vi "ReadArrayDouble(DBL).vi"(8 "error in (no error)":errorcluster, 9 "Elements (-1 = auto)":i32, 10 "variableName":string, 11 "TCatAdsNet in":refnum<class "AdsNET.lvclass">) -> (0 "error out":errorcluster, 2 "Values (DBL)":dbl[](array[numeric]), 3 "TCatAdsNet out":refnum<class "AdsNET.lvclass">)   [LabVIEW 2016, in "TCatAdsNet.lvlib" / "AdsNET.lvclass"]
uses:
  AdsNET.lvclass
  AdsNET.lvclass/AdsNET.ctl
  C:/Users/Maurizio/Projects/twincat-lv-ads-library/TCatAdsNet Library/TwinCAT.Ads.dll
  TwinCAT.Ads.dll
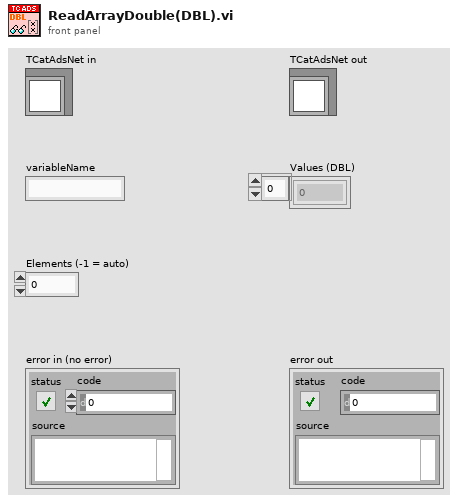
[diagram p1: front panel]
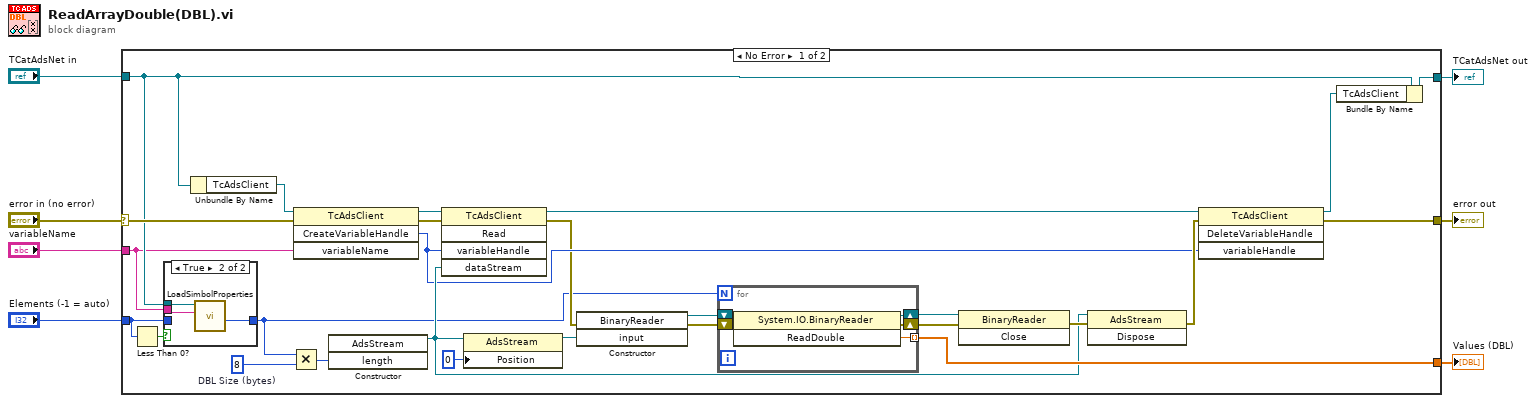
[diagram p0: block diagram]
diagram:
  n1 = case shown="No Error" "error in (no error)" {
    selector: "error in (no error)" -> [w13 w43]
    tunnel: [w27 _] -> w7
    tunnel: "variableName" -> [w10 _]
    tunnel: "Elements (-1 = auto)" -> [w9 _]
    tunnel: [w16 w44] -> w4
    tunnel: [w14 w43] -> w3
    tunnel: "TCatAdsNet in" -> [w11 w44]
    frame No Error {
      w32 = 8  # DBL Size (bytes)
      n2 = Less Than 0?(x=w9) -> (x < 0?=w8:bool)
      n3 = case shown="True" w8 {
        tunnel: w9 -> [w35 _]
        tunnel: [w35 w38] -> w12
        tunnel: w11 -> [_ w37]
        tunnel: w10 -> [_ w36]
        frame False {
        }
        frame True {
          n4 = call "LoadSimbolProperties.vi"("name"=w36, "TCatAdsNet in"=w37) -> ("Elements"=w38:i32)  [unwired: 6 in, 3 out]
        }
      }
      n5 = Unbundle By Name(w11) -> ("TcAdsClient"=w17:refnum<k24>)
      n6 = Multiply ("Multiplizieren")(x=w12, y=w32) -> (x*y=w31:i32)
      n7 = invoke class="TcAdsClient" method="CreateVariableHandle"(reference=w17, error in=w13, "variableName"=w10) -> (reference out=w34:refnum<k24>, error out=w33:errorcluster, "CreateVariableHandle"=w19:i32)  [unwired: 1 in, 1 out]
      n8 = constructor class="AdsStream" ("Konstruktorknoten")("length"=w31) -> (reference out=w21:refnum<k24>)  [unwired: 3 in, 3 out]
      n9 = invoke class="TcAdsClient" method="Read"(reference=w34, error in=w33, "variableHandle"=w19, "dataStream"=w21) -> (reference out=w22:refnum<k24>, error out=w18:errorcluster)  [unwired: 1 in, 3 out]
      n10 = property class="AdsStream"(reference=w21, "Position"=i64 0) -> (reference out=w29:refnum<k24>)  [unwired: 1 in, 1 out]
      n11 = constructor class="BinaryReader"(error in=w18, "input"=w29) -> (reference out=w28:refnum<k24>, error out=w25:errorcluster)  [unwired: 2 in, 2 out]
      n12 = for {
        N: w12 -> [_]
        tunnel: [w41] -> w27 mode=indexing
        shift-right: [w40] -> w26
        shift-left: w28 -> [w42]
        shift-right: [w39] -> w24
        shift-left: w25 -> [_]
        n13 = invoke class="System.IO.BinaryReader" method="ReadDouble"(reference=w42) -> (reference out=w40:refnum<k24>, error out=w39:errorcluster, "ReadDouble"=w41:dbl)  [unwired: 2 in]
      }
      n14 = invoke class="BinaryReader" method="Close"(reference=w26, error in=w24) -> (error out=w23:errorcluster)  [unwired: 1 in, 2 out]
      n15 = invoke class="AdsStream" method="Dispose"(reference=w21, error in=w23) -> (error out=w20:errorcluster)  [unwired: 1 in, 2 out]
      n16 = invoke class="TcAdsClient" method="DeleteVariableHandle"(reference=w22, error in=w20, "variableHandle"=w19) -> (reference out=w15:refnum<k24>, error out=w14:errorcluster)  [unwired: 1 in, 2 out]
      n17 = Bundle By Name(cluster=w11, "TcAdsClient"=w15) -> (w16:refnum<class "AdsNET.lvclass">)
    }
    frame Error {
    }
  }
  "TCatAdsNet out" <- w4
  "Values (DBL)" <- w7
  "error out" <- w3
